vi "demo.vi"() -> ()   [LabVIEW 2020]
uses:
  <vilib>/PantherLAB/Firebase API/PantherLAB_lib_Filtering Parameters--cluster.ctl
  38fb2073-e18a-44cf-a881-8404aca7a24e.vi
  04e791fb-3a71-4957-a507-870e153ef2ab.vi
  66751dfa-5380-4681-ab0e-58deb68600d4.vi
  <vilib>/JDP Science/JSONtext/JSON text to Variant.vi
  <vilib>/JDP Science/JSONtext/LVClass Serializer/JSONtext LVClass Serializer.lvclass
  <vilib>/PantherLAB/Firebase API/PantherLAB_lib_firebase.lvclass
  <vilib>/JDP Science/JSONtext/JSONtext.lvlib
panel:
  in  "Exit":bool
  in  "Tab Control":enum32{"Log IN/Sign IN", "POST", "GET", "PUT"}(tab)
  in  "Password":string
  in  "Email":string
  in  "Log In":bool
  in  "Sign In":bool
  in  "Volts":dbl(knob) scale=0.0..1000.0
  in  "Enable":bool
  in  "Post":bool
  out "data":T1 {"date" format="%<%x %.3X>T"}
  in  "Get Newest":bool
  out "Elements":T2(array[cluster]) {"date" format="%<%x %.3X>T"}
  in  "Get Last 5":bool
  out "JSON String":string
  in  "Delete":bool
  in  "Get All":bool
  in  "Date":timestamp
  in  "Amperes":dbl(knob) scale=0.0..1000.0
  in  "Light":bool
  in  "PUT":bool
  # "To add an authenticated user\nto your Real Time Database"
  # "If you are already authenticated\nand you want to start using\nyour Database"
  # "Use Post if you want to create a new Database Item Each Time"
  # "Warning:\nThis button will delete all the data\nunder data endpoint"
  # "Use PUT  if you want to override a  Database Item"
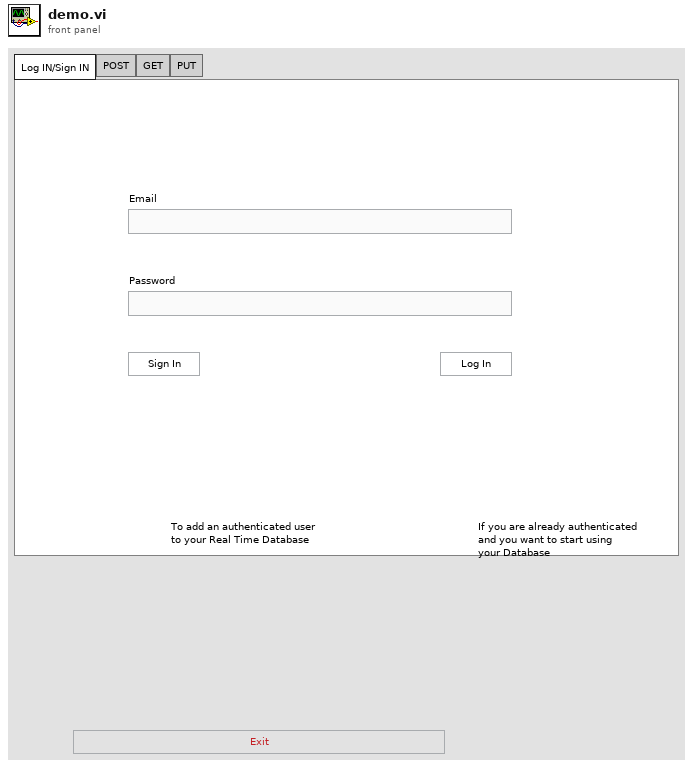
[diagram p1: front panel]
types:
  T1 = cluster{"Volts":dbl, "Enable":bool, "date":timestamp}
  T2 = cluster{"Volts":dbl, "Enable":bool, "date":timestamp}[]
  T3 = typedef "PantherLAB_lib_firebase.lvclass/PantherLAB_lib_Filtering Parameters--cluster.ctl" = cluster{"Filtering Param":string, "Argument":string}
  T4 = cluster{"Amperes":dbl, "Light":bool, "Date":timestamp}
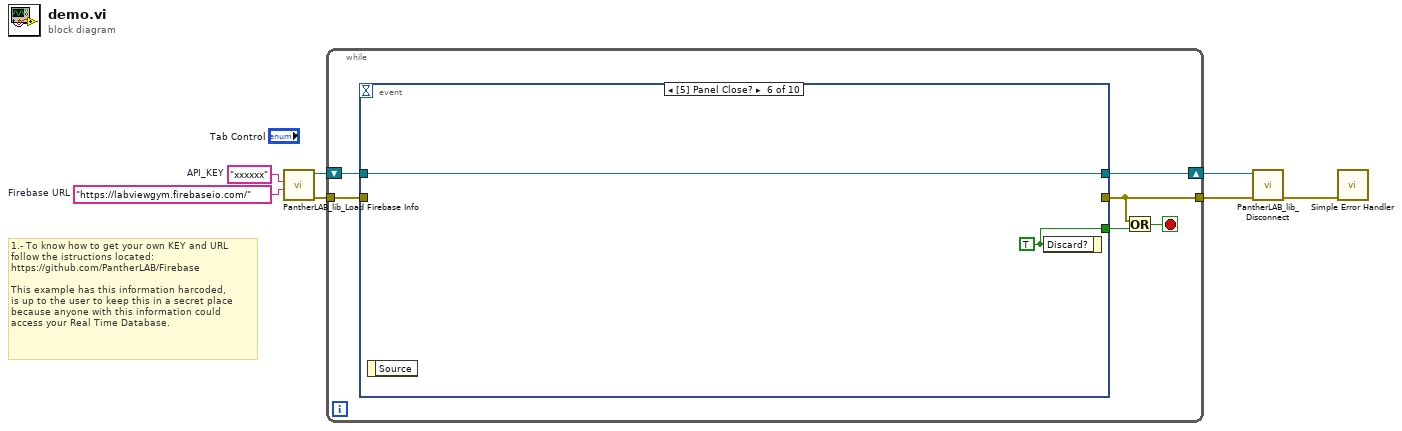
[diagram p0: block diagram]
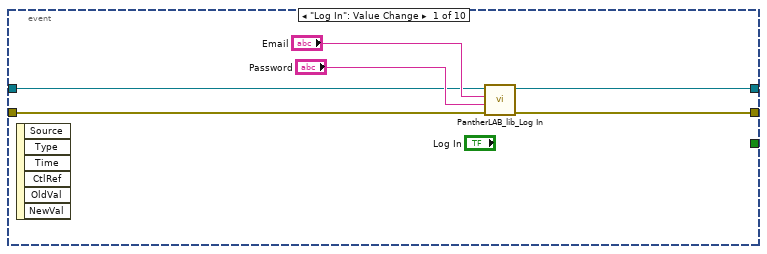
[diagram p2: hidden frame]
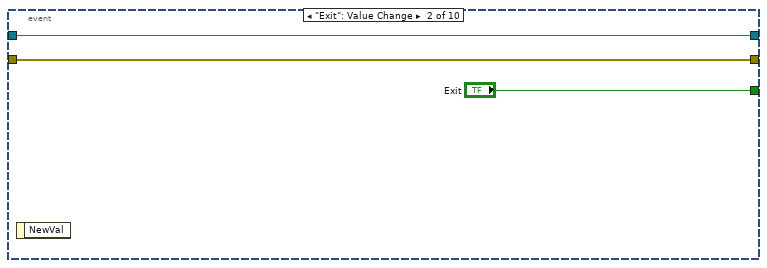
[diagram p3: hidden frame]
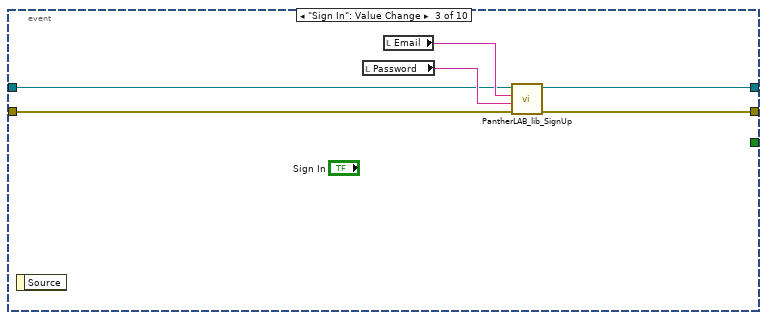
[diagram p4: hidden frame]
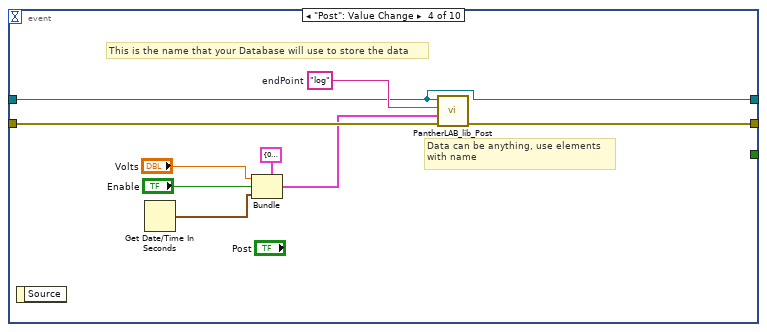
[diagram p5: hidden frame]
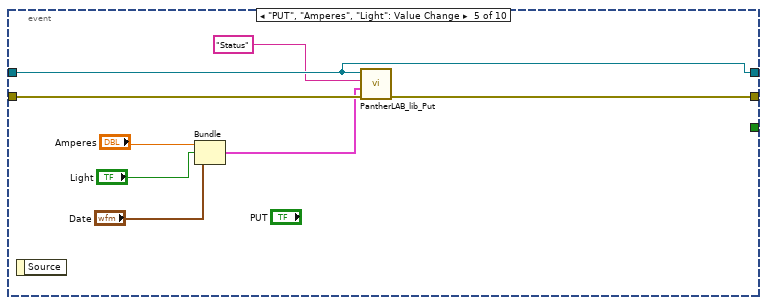
[diagram p6: hidden frame]
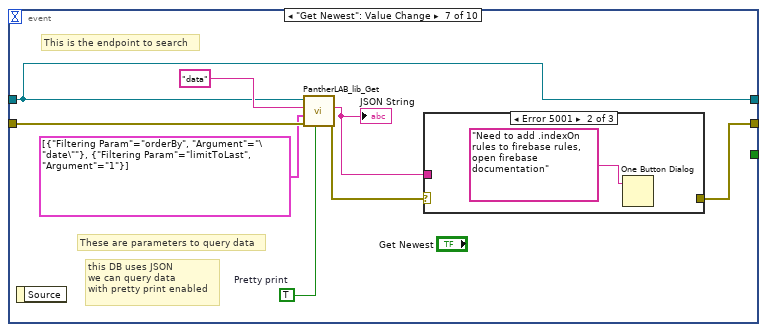
[diagram p7: hidden frame]
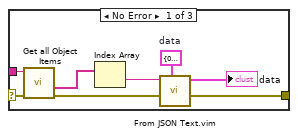
[diagram p8: hidden frame]
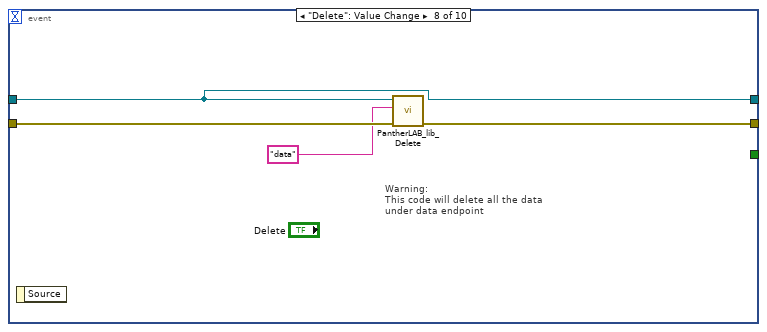
[diagram p10: hidden frame]
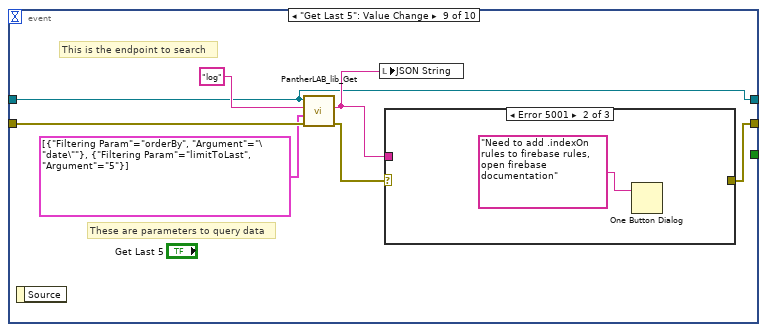
[diagram p11: hidden frame]
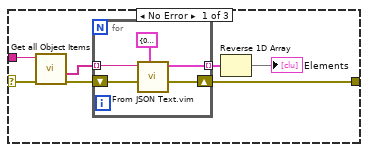
[diagram p12: hidden frame]
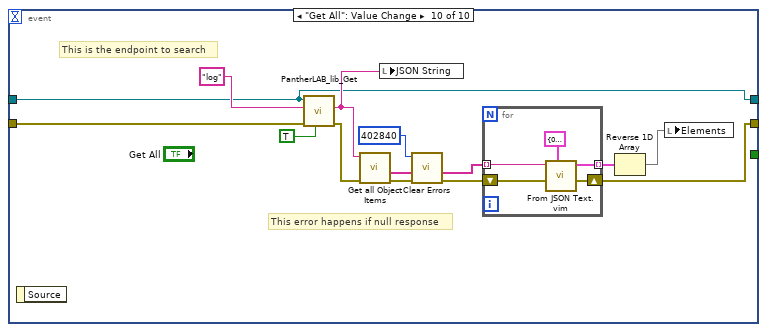
[diagram p14: hidden frame]
diagram:
  w2 = "xxxxxx"  # API_KEY
  w1 = "https://labviewgym.firebaseio.com/"  # Firebase URL
  # "1.- To know how to get your own KEY and URL\nfollow the istructions located:\nhttps://github.com/PantherLAB/Firebase\n\nThis example has this information harcoded,\nis up to the user to keep this in a secret place\nbecause anyone with this information could\naccess your Real Time Database."
  n1 = call <vilib>:"PantherLAB_lib_Load Firebase Info.vi"("Firebase URL"=w1, "API_KEY"=w2) -> ("error out"=w5:errorcluster, "firebase out"=w3:refnum<class "PantherLAB_lib_firebase.lvclass">)  [unwired: 8 in]
  n2 = while {
    tunnel: w5 -> [w13]
    tunnel: [w12] -> w6
    shift-right: [w8] -> w4
    shift-left: w3 -> [w9]
    stop <- w10 stop-if-true
    n3 = event shown="[5] Panel Close?" {
      selector: _ -> [_ _ _ _ _ _ _ _ _ _]
      dyn-events: _ -> [_ _ _ _ _ _ _ _ _ _]
      timeout: _ -> [_ _ _ _ _ _ _ _ _ _]
      tunnel: w13 -> [w19 w22 w28 w37 w45 _ w55 w69 w76 w103]
      tunnel: [w18 w22 w27 w36 w44 _ w53 w68 w74 w100] -> w12
      tunnel: [_ "Exit" _ _ _ w46 _ _ _ _] -> w11
      tunnel: w9 -> [w15 w20 w24 w29 w43 w47 w48 w66 w70 w91]
      tunnel: [w14 w20 w23 w29 w43 w47 w48 w66 w70 w91] -> w8
      event "Log In": Value Change {
        n4 = event-data() -> ()  [unwired: 1 in, 6 out]
        n5 = call-dynamic "PantherLAB_lib_Log In.vi"("error in"=w19, "password"="Password", "email"="Email", "firebase in"=w15) -> ("error out"=w18:errorcluster, "firebase out"=w14:refnum<class "PantherLAB_lib_firebase.lvclass">)  [unwired: 6 in]
      }
      event "Exit": Value Change {
        n6 = event-data() -> ()  [unwired: 1 in, 1 out]
      }
      event "Sign In": Value Change {
        n7 = event-data() -> ()  [unwired: 1 in, 1 out]
        n8 = local read "Password"() -> (w26:string)
        n9 = local read "Email"() -> (w25:string)
        n10 = call-dynamic "PantherLAB_lib_SignUp.vi"("error in"=w28, "password"=w26, "email"=w25, "firebase in"=w24) -> ("error out"=w27:errorcluster, "firebase out"=w23:refnum<class "PantherLAB_lib_firebase.lvclass">)  [unwired: 6 in]
      }
      event "Post": Value Change {
        w35 = "log"  # endPoint
        # "This is the name that your Database will use to store the data"
        # "Data can be anything, use elements\nwith name"
        n11 = event-data() -> ()  [unwired: 1 in, 1 out]
        n12 = Get Date/Time In Seconds() -> (seconds since 1Jan1904=w34:timestamp)
        n13 = Bundle(cluster=T1 {"Volts"=0.0, "Enable"=FALSE, "date"=timestamp(0 s since 1904-01-01)}, "Volts"="Volts", "Enable"="Enable", "date"=w34) -> (w33:T1)
        n14 = call-dynamic "PantherLAB_lib_Post.vi"("error in"=w37, "Anything"=w33, "endPoint"=w35, "firebase in"=w29) -> ("error out"=w36:errorcluster)  [unwired: 6 in, 1 out]
      }
      event "PUT", "Amperes", "Light": Value Change {
        n15 = event-data() -> ()  [unwired: 1 in, 1 out]
        n16 = Bundle("Amperes"="Amperes", "Light"="Light", "Date"="Date") -> (w38:T4)  [unwired: 1 in]
        n17 = call-dynamic "PantherLAB_lib_Put.vi"("error in"=w45, "Anything"=w38, "endPoint"="Status", "firebase in"=w43) -> ("error out"=w44:errorcluster)  [unwired: 6 in, 1 out]
      }
      event Panel Close? {
        w46 = TRUE ("Discard?")
        n18 = event-data() -> ()  [unwired: 1 in, 1 out]
        n19 = event-data("Discard?"=w46) -> ()  [unwired: 1 in, 1 out]
      }
      event "Get Newest": Value Change {
        w49 = TRUE  # Pretty print
        # "this DB uses JSON\nwe can query data\nwith pretty print enabled"
        # "These are parameters to query data"
        # "This is the endpoint to search"
        n20 = event-data() -> ()  [unwired: 1 in, 1 out]
        n21 = call-dynamic "PantherLAB_lib_Get.vi"("Pretty print"=w49, "error in"=w55, "Filtering Params"=T3[] [{"Filtering Param"="orderBy", "Argument"="\"date\""}, {"Filtering Param"="limitToLast", "Argument"="1"}], "endPoint"="data", "firebase in"=w48) -> ("error out"=w54:errorcluster, "Json String"=w50:string)  [unwired: 5 in]
        "JSON String" <- w50
        n22 = case shown="Error 5001" w54 {
          selector: w54 -> [w63 _ w65]
          tunnel: [w61 _ w65] -> w53
          tunnel: w50 -> [w57 _ _]
          frame No Error {
            w60 = T1 {"Volts"=0.0, "Enable"=FALSE, "date"=timestamp(0 s since 1904-01-01)}  # data
            n23 = call <vilib>:"Get all Object Items.vi"("error in (no error)"=w63, "JSON"=w57) -> ("error out"=w62:errorcluster, "<JSON>"=w59:string[])  [unwired: 6 in, 2 out]
            n24 = Index Array(array=w59) -> (element=w58:string)  [unwired: 1 in]
            n25 = call "From JSON Text.vim"("Data Type and Default Value"=w60, "error in (no error)"=w62, "JSON"=w58) -> ("error out"=w61:errorcluster, "Data out"=→"data":T1)  [unwired: 7 in]
          }
          frame Error {
            n26 = One Button Dialog(message="Need to add .indexOn rules to firebase rules, open firebase documentation") -> ()  [unwired: 1 in, 1 out]
          }
          frame Default {
          }
        }
      }
      event "Delete": Value Change {
        # "Warning:\nThis code will delete all the data\nunder data endpoint"
        n27 = event-data() -> ()  [unwired: 1 in, 1 out]
        n28 = call-dynamic "PantherLAB_lib_Delete.vi"("error in"=w69, "endPoint"="data", "firebase in"=w66) -> ("error out"=w68:errorcluster)  [unwired: 7 in, 1 out]
      }
      event "Get Last 5": Value Change {
        # "This is the endpoint to search"
        # "These are parameters to query data"
        n29 = event-data() -> ()  [unwired: 1 in, 1 out]
        n30 = call-dynamic "PantherLAB_lib_Get.vi"("error in"=w76, "Filtering Params"=T3[] [{"Filtering Param"="orderBy", "Argument"="\"date\""}, {"Filtering Param"="limitToLast", "Argument"="5"}], "endPoint"="log", "firebase in"=w70) -> ("error out"=w75:errorcluster, "Json String"=w71:string)  [unwired: 6 in]
        n31 = local write "JSON String"(w71) -> ()
        n32 = case shown="Error 5001" w75 {
          selector: w75 -> [w82 _ w90]
          tunnel: [w81 _ w90] -> w74
          tunnel: w71 -> [w77 _ _]
          frame No Error {
            n33 = call <vilib>:"Get all Object Items.vi"("error in (no error)"=w82, "JSON"=w77) -> ("error out"=w83:errorcluster, "<JSON>"=w80:string[])  [unwired: 6 in, 2 out]
            n34 = for {
              tunnel: w80 -> [w85] mode=indexing
              shift-right: [w87] -> w81
              shift-left: w83 -> [w88]
              tunnel: [w84] -> w79 mode=indexing
              n35 = call "From JSON Text.vim"("Data Type and Default Value"=T1 {"Volts"=0.0, "Enable"=FALSE, "date"=timestamp(0 s since 1904-01-01)} ("data"), "error in (no error)"=w88, "JSON"=w85) -> ("error out"=w87:errorcluster, "Data out"=w84:T1)  [unwired: 7 in]
            }
            n36 = Reverse 1D Array(array=w79) -> (reversed array=→"Elements":T2)
          }
          frame Error {
            n37 = One Button Dialog(message="Need to add .indexOn rules to firebase rules, open firebase documentation") -> ()  [unwired: 1 in, 1 out]
          }
          frame Default {
          }
        }
      }
      event "Get All": Value Change {
        # "This error happens if null response"
        # "This is the endpoint to search"
        n38 = event-data() -> ()  [unwired: 1 in, 1 out]
        n39 = call-dynamic "PantherLAB_lib_Get.vi"("Pretty print"=TRUE, "error in"=w103, "endPoint"="log", "firebase in"=w91) -> ("error out"=w101:errorcluster, "Json String"=w95:string)  [unwired: 6 in]
        n40 = call <vilib>:"Get all Object Items.vi"("error in (no error)"=w101, "JSON"=w95) -> ("error out"=w102:errorcluster, "<JSON>"=w97:string[])  [unwired: 6 in, 2 out]
        n41 = local write "JSON String"(w95) -> ()
        n42 = call <vilib>:"Clear Errors.vi"("error in (no error)"=w102, "specific error code to clear (0: all)"=402840) -> ("error out"=w99:errorcluster)  [unwired: 4 in, 1 out]
        n43 = for {
          tunnel: w97 -> [w105] mode=indexing
          shift-right: [w107] -> w100
          shift-left: w99 -> [w108]
          tunnel: [w104] -> w96 mode=indexing
          n44 = call "From JSON Text.vim"("Data Type and Default Value"=T1 {"Volts"=0.0, "Enable"=FALSE, "date"=timestamp(0 s since 1904-01-01)} ("data"), "error in (no error)"=w108, "JSON"=w105) -> ("error out"=w107:errorcluster, "Data out"=w104:T1)  [unwired: 7 in]
        }
        n45 = Reverse 1D Array(array=w96) -> (reversed array=w94:T2)
        n46 = local write "Elements"(w94) -> ()
      }
    }
    n47 = Or(x=w12, y=w11) -> (x .or. y?=w10:bool)
  }
  n48 = call-dynamic "PantherLAB_lib_Disconnect.vi"("error in"=w6, "firebase in"=w4) -> ("error out"=w7:errorcluster)  [unwired: 9 in]
  n49 = call <vilib>:"Simple Error Handler.vi"("error in (no error)"=w7) -> ()  [unwired: 4 in, 5 out]
